vi "_Open SequenceFile.vi"(7 "File Load Options":T1={"Use Search Dirs? (T)"=TRUE, "Conflict as Error? (T)"=TRUE, "Check Station Model? (F)"=FALSE, "Preload Modules? (T)"=TRUE, "Skip Load Callback? (F)"=FALSE, "Reload if Loaded? (F)"=FALSE}, 9 "Current SeqFile":refnum<class "SequenceFile.lvclass">, 10 "File Path":path, 11 "Engine in":refnum<class "Engine.lvclass">) -> (0 "error out":errorcluster, 2 "SequenceFile":refnum<class "SequenceFile.lvclass">)   [LabVIEW 2020, in "TSnax.lvlib" / "Engine.lvclass"]
uses:
  Engine.lvclass
  Engine.lvclass/Engine.ctl
  SequenceFile/SequenceFile.lvclass
  SequenceFile/File Load Options.ctl
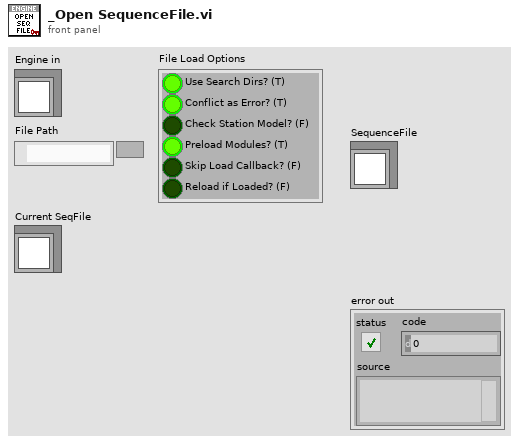
[diagram p1: front panel]
types:
  T1 = typedef "TSnax.lvlib/SequenceFile.lvclass/File Load Options.ctl" = cluster{"Use Search Dirs? (T)":bool, "Conflict as Error? (T)":bool, "Check Station Model? (F)":bool, "Preload Modules? (T)":bool, "Skip Load Callback? (F)":bool, "Reload if Loaded? (F)":bool}
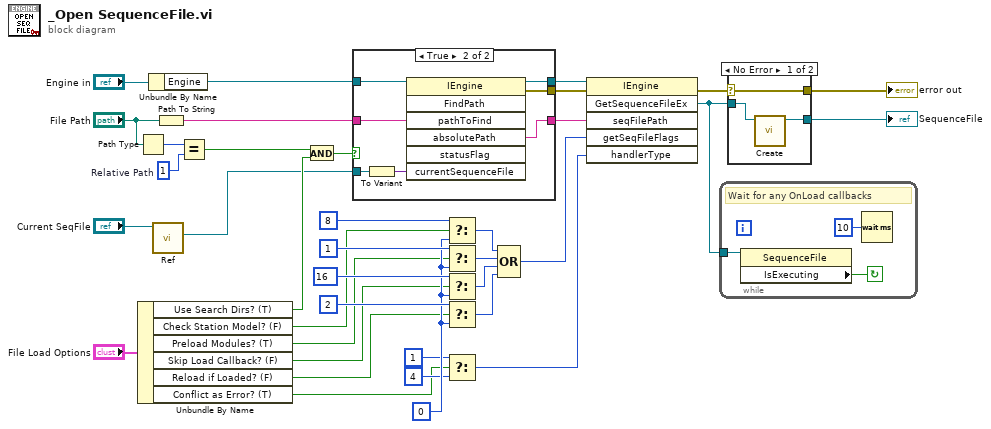
[diagram p0: block diagram]
diagram:
  w19 = i16 1  # Relative Path
  w33 = 0 ("getSeqFileFlags")
  n1 = Path Type(1:"File Path") -> (0:w20:i16)
  n2 = Unbundle By Name("File Load Options") -> ("Use Search Dirs? (T)"=w16:bool, "Check Station Model? (F)"=w25:bool, "Preload Modules? (T)"=w24:bool, "Skip Load Callback? (F)"=w23:bool, "Reload if Loaded? (F)"=w22:bool, "Conflict as Error? (T)"=w21:bool)
  n3 = Unbundle By Name("Engine in") -> ("Engine"=w12:refnum<k7>)
  n4 = call "Ref.vi"("SequenceFile in"="Current SeqFile") -> ("Ref"=w1:refnum<k7>)  [unwired: 8 in, 2 out]
  n5 = Path To String(path="File Path") -> (string=w14:string)
  n6 = Equal?(x=w20, y=w19) -> (x = y?=w17:bool)
  n7 = And(x=w17, y=w16) -> (x .and. y?=w15:bool)
  n8 = case shown="True" w15 {
    tunnel: w14 -> [w39 w46]
    tunnel: w12 -> [w38 w44]
    tunnel: [w39 w43] -> w9
    tunnel: [w38 w42] -> w11
    tunnel: [_ w41] -> w10
    tunnel: w1 -> [_ w40]
    frame False {
    }
    frame True {
      n9 = To Variant(anything=w40) -> (Variant=w45:variant)
      n10 = invoke class="IEngine" method="FindPath"(reference=w44, "pathToFind"=w46, "currentSequenceFile"=w45) -> (reference out=w42:refnum<k7>, error out=w41:errorcluster, "absolutePath"=w43:string)  [unwired: 4 in, 4 out]
    }
  }
  n11 = Select(t=8 ("getSeqFileFlags"), s=w25, f=w33) -> (s? t:f=w29:i32)
  n12 = Select(t=1 ("getSeqFileFlags"), s=w24, f=w33) -> (s? t:f=w30:i32)
  n13 = Select(t=16 ("getSeqFileFlags"), s=w23, f=w33) -> (s? t:f=w28:i32)
  n14 = Select(t=2 ("getSeqFileFlags"), s=w22, f=w33) -> (s? t:f=w27:i32)
  n15 = Select(t=1 ("getSeqFileFlags"), s=w21, f=4 ("getSeqFileFlags")) -> (s? t:f=w7:i32)
  n16 = Compound Arithmetic op=OR(w29, w30, w28, w27) -> (w8:i32)
  n17 = invoke class="IEngine" method="GetSequenceFileEx"(reference=w11, error in=w10, "seqFilePath"=w9, "getSeqFileFlags"=w8, "handlerType"=w7) -> (error out=w5:errorcluster, "GetSequenceFileEx"=w6:refnum<k7>)  [unwired: 1 in, 4 out]
  n18 = while {
    tunnel: w6 -> [w49]
    stop <- w48 continue-if-true
    # "Wait for any OnLoad callbacks"
    n19 = property class="SequenceFile"(reference=w49) -> ("IsExecuting"=w48:bool)  [unwired: 1 in, 2 out]
    n20 = Wait (ms)(milliseconds to wait=u32 10) -> ()  [unwired: 1 out]
  }
  n21 = case shown="No Error" w5 {
    selector: w5 -> [w51 w53]
    tunnel: w6 -> [w52 _]
    tunnel: [w51 w53] -> w4
    tunnel: [w50 _] -> w3
    frame No Error {
      n22 = call "Create.vi"("SequenceFile"=w52) -> ("SequenceFile out"=w50:refnum<class "SequenceFile.lvclass">)  [unwired: 9 in, 1 out]
    }
    frame Error {
    }
  }
  "error out" <- w4
  "SequenceFile" <- w3
